vi "数据读取.vi"(0 "字符串":string) -> (1 "ADC":u16, 2 "ENC":u16)   [LabVIEW 2022 SP3]
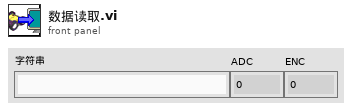
[diagram p1: front panel]
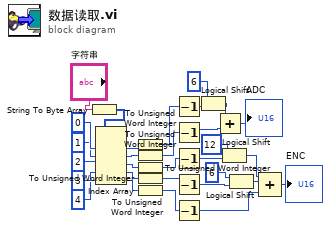
[diagram p0: block diagram]
diagram:
  n1 = String To Byte Array(string="字符串") -> (unsigned byte array=w14:u8[])
  n2 = Index Array(array=w14, index #1=0 ("索引"), index #2=1 ("索引"), index #3=2 ("索引"), index #4=3 ("索引"), index #5=4 ("索引")) -> (element #1=w11:u8, element #2=w21:u8, element #3=w24:u8, element #4=w25:u8, element #5=w26:u8)
  n3 = To Unsigned Word Integer(number=w11) -> (unsigned 16bit integer=w10:u16)
  n4 = To Unsigned Word Integer(number=w21) -> (unsigned 16bit integer=w22:u16)
  n5 = To Unsigned Word Integer(number=w24) -> (unsigned 16bit integer=w27:u16)
  n6 = To Unsigned Word Integer(number=w25) -> (unsigned 16bit integer=w28:u16)
  n7 = To Unsigned Word Integer(number=w26) -> (unsigned 16bit integer=w29:u16)
  n8 = Decrement(x=w10) -> (x-1=w9:u16)
  n9 = Decrement(x=w22) -> (x-1=w23:u16)
  n10 = Decrement(x=w27) -> (x-1=w5:u16)
  n11 = Decrement(x=w28) -> (x-1=w3:u16)
  n12 = Decrement(x=w29) -> (x-1=w30:u16)
  n13 = Logical Shift(y=i16 6, x=w9) -> (x << y=w7:u16)
  n14 = Add(x=w7, y=w23) -> (x+y=→"ADC":u16)
  n15 = Logical Shift(y=i16 12, x=w5) -> (x << y=w6:u16)
  n16 = Logical Shift(y=i16 6, x=w3) -> (x << y=w1:u16)
  n17 = Compound Arithmetic op=ADD(w6, w1, w30) -> (→"ENC":u16)
